vi "Initialize.vi"   [LabVIEW 2011, in "PolarVector.lvclass"]
uses:
  PolarVector.lvclass
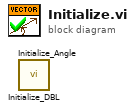
[diagram p0: block diagram]
diagram:
  n1 = call "Initialize_DBL.vi"() -> ()  [unwired: 10 in, 2 out]
  n2 = call "Initialize_Angle.vi"() -> ()  [unwired: 10 in, 2 out]
